vi "GFITS_AddKeyword.vi"(5 "auxhdr":path=path "", 7 "Database RefNum":T1, 8 "error in":errorcluster, 11 "command in":string) -> (0 "error out":errorcluster)   [LabVIEW 2016]
uses:
  DBSHAND/private/vis/DatabaseHand_RefNum.ctl
  GFITS_Gbls.vi
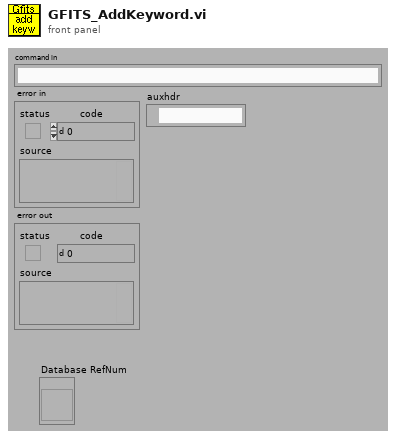
[diagram p1: front panel]
types:
  T1 = typedef "DatabaseHand_RefNum.ctl" = refnum<vi>
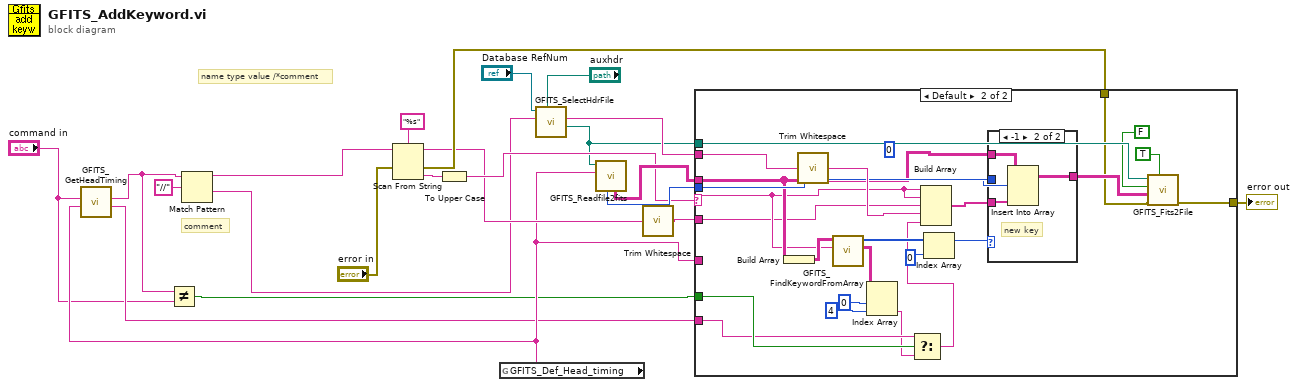
[diagram p0: block diagram]
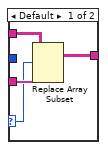
[diagram p3: hidden frame]
diagram:
  # "comment"
  # "name type value /*comment"
  n1 = global read "GFITS_Gbls.vi" "GFITS_Def_Head_timing"() -> (w5:string)
  n2 = call "GFITS_GetHeadTiming.vi"("def_timing"=w5, "line In"="command in") -> ("head_tim"=w4:string, "line out"=w3:string)  [unwired: 8 out]
  n3 = Not Equal?(x=w3, y="command in") -> (x != y?=w1:bool)
  n4 = Match Pattern(string=w3, regular expression="//") -> (before substring=w13:string, after substring=w9:string)  [unwired: 3 out]
  n5 = Scan From String(format string="%s" ("Format String"), input string=w13, error in="error in") -> (remaining string=w12:string, error out=w18:errorcluster, output 1=w21:string)  [unwired: 1 in, 2 out]
  n6 = To Upper Case(1:w21) -> (0:w14:string)
  n7 = call "GFITS_SelectHdrFile.vi"("auxhdr"="auxhdr", "line in"=w9, "Database RefNum"="Database RefNum") -> ("path out"=w7:path, "line out"=w8:string)  [unwired: 7 out]
  n8 = call "GFITS_Readfile2fits.vi"("def_timing"=w5, "file"=w7) -> ("all keys"=w17:string[][], "number of total keywords"=w16:i32)  [unwired: 8 out]
  n9 = call <vilib>:"Trim Whitespace.vi"("string"=w12) -> ("trimmed string"=w11:string)  [unwired: 1 in]
  n10 = case shown="Default" w14 {
    selector: w14 -> [_ w37]
    tunnel: w17 -> [_ w42]
    tunnel: w7 -> [_ w46]
    tunnel: w16 -> [_ w43]
    tunnel: [w23 w36] -> w19
    tunnel: w18 -> [w23 w35]
    tunnel: w8 -> [_ w31]
    tunnel: w11 -> [_ w28]
    tunnel: w5 -> [_ _]
    tunnel: w4 -> [_ w26]
    tunnel: w1 -> [_ w27]
    frame "", " " {
    }
    frame Default {
      (unwired) 0 ("Index (page)")
      n11 = Build Array(w42) -> (w41:string[][][])
      n12 = call <vilib>:"Trim Whitespace.vi"("string"=w31) -> ("trimmed string"=w47:string)  [unwired: 1 in]
      n13 = call "GFITS_FindKeywordFromArray.vi"("Keyword"=w37, "Keywords"=w41) -> ("values"=w34:string[][], "indexes"=w40:i16[])  [unwired: 8 out]
      n14 = Index Array(array=w34, index (row)=0, index (col)=4 ("disabled index (col)")) -> (element=w25:string)
      n15 = Select(t=w26, s=w27, f=w25) -> (s? t:f=w24:string)
      n16 = Build Array(w37, w37, w28, w47, w24) -> (w45:string[])
      n17 = Index Array(array=w40, index=0 ("Index")) -> (element=w38:i16)
      n18 = case shown="-1" w38 {
        selector: w38 -> [w49 _]
        tunnel: w45 -> [w50 w55]
        tunnel: [w48 w54] -> w44
        tunnel: w43 -> [_ w53]
        tunnel: w42 -> [w51 w52]
        frame Default {
          n19 = Replace Array Subset(array=w51, new element=w50, index (row)=w49) -> (w48:string[][])  [unwired: 1 in]
        }
        frame -1 {
          # "new key"
          n20 = Insert Into Array(array=w52, index (row)=w53, new element=w55) -> (w54:string[][])  [unwired: 1 in]
        }
      }
      n21 = call "GFITS_Fits2File.vi"("write to file?"=TRUE, "error in (no error)"=w35, "Keywords"=w44, "append to file? (new file:F)"=FALSE, "filename"=w46) -> ("error out"=w36:errorcluster)  [unwired: 6 out]
    }
  }
  "error out" <- w19
